vi "LVH5AreadUnitsArray.vi"(6 "error in (no error)":errorcluster, 8 "Name":string, 9 "HDF5 Location in":T1) -> (0 "error out":errorcluster, 1 "Value":T2[](array[typedef]), 3 "HDF5 Location out":T1)   [LabVIEW 2017]
doc: "This is a high level VI for writing string attributes only. It should not normally need to be called by users of LVHDF5. They should instead call Simple H5Awrite. This was implemented to break a recursion cycle in Type Caching."
uses:
  <vilib>/Utility/VariantDataType/UnitInfo.ctl
  <vilib>/Utility/VariantDataType/UnitType.ctl
  <vilib>/UPVI/lvhdf5/library.llb/HDF5 Ref.ctl
  <vilib>/Utility/VariantDataType/VariantType.lvlib
  <vilib>/UPVI/lvhdf5/h5helper.dll
panel:
  # "LVHDF5 Toolkit\nCopyright (c) 2005-2013 by Jason D. Sommerville\nCopyright (c) 2014 by UPVI, LLC.\n\nThis use and distribution of this file is governed by the terms found in \nLICENSE.txt distributed with this toolkit and installed at\n <user.lib>\\_lvhdf5\\LICENSE.txt"
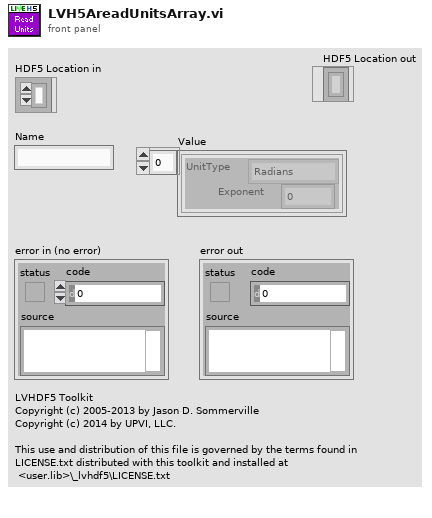
[diagram p1: front panel]
types:
  T1 = typedef "HDF5 Ref.ctl" = refnum<k1>
  T2 = typedef "VariantType.lvlib/UnitInfo.ctl" = cluster{"UnitType":T3, "Exponent":i16}
  T3 = typedef "VariantType.lvlib/UnitType.ctl" = enum16{"Radians", "Steradians", "Seconds", "Meters", "Kilograms", "Amperes", "Kelvins", "Moles", "Candelas", "InvalidUnit"}
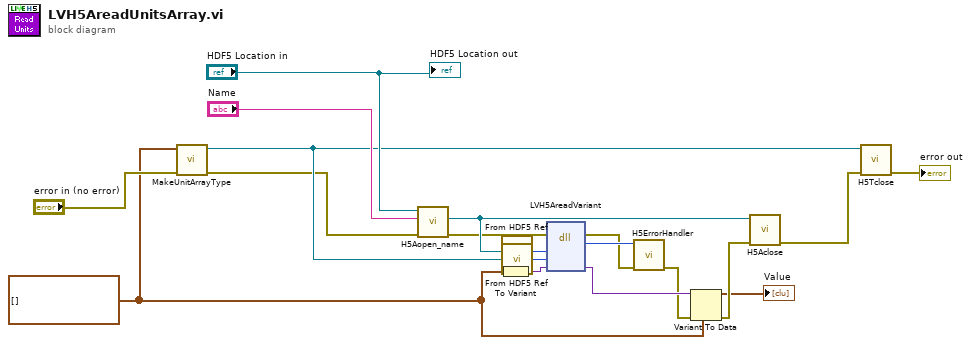
[diagram p0: block diagram]
diagram:
  w1 = T2[] [] ("Value")
  n1 = call <vilib>:"MakeUnitArrayType.vi"("error in (no error)"="error in (no error)", "Unit Array"=w1) -> ("error out"=w8:errorcluster, "Refnum out"=w9:T1)  [unwired: 8 in]
  n2 = call <vilib>:"H5Aopen_name.vi"("error in (no error)"=w8, "name"="Name", "HDF5 Ref"="HDF5 Location in") -> ("error out"=w12:errorcluster, "HDF5 Attr Ref"=w13:T1)  [unwired: 4 in, 1 out]
  n3 = To Variant(anything=w1) -> (Variant=w6:variant)
  n4 = call <vilib>:"From HDF5 Ref.vi"("HDF5 Ref"=w13) -> ("I32"=w19:i32)
  n5 = call <vilib>:"From HDF5 Ref.vi"("HDF5 Ref"=w9) -> ("I32"=w18:i32)
  n6 = dll-call lib="C:/Program Files/National Instruments/LabVIEW 2017/vi.lib/UPVI/lvhdf5/h5helper.dll" fn="LVH5AreadVariant" label="LVH5AreadIndirect"(error in=w12, "attr_id"=w19, "mem_type_id"=w18, "Value"=w6) -> (error out=w14:errorcluster, "return type"=w15:i32, "Value"=w5:variant)  [unwired: 4 in, 1 out]
  n7 = call <vilib>:"H5ErrorHandler.vi"("error in (no error)"=w14, "herr_t"=w15) -> ("error out"=w4:errorcluster)  [unwired: 3 in, 4 out]
  n8 = Variant To Data(error in=w4, type=w1, Variant=w5) -> (data=→"Value":T2[], error out=w3:errorcluster)
  n9 = call <vilib>:"H5Aclose.vi"("error in (no error)"=w3, "HDF5 Dataset Ref"=w13) -> ("error out"=w7:errorcluster)  [unwired: 7 in]
  n10 = call <vilib>:"H5Tclose.vi"("error in (no error)"=w7, "HDF5 Datatype Ref"=w9) -> ("error out"=→"error out":errorcluster)  [unwired: 7 in]
  "HDF5 Location out" <- "HDF5 Location in"
